vi "Lift Safety.vi"(11 "Operation States":T2) -> (3 "Operation States Out":T2)   [LabVIEW 2014]
uses:
  <vilib>/Rock Robotics/WPI/Solenoid/WPI_SolenoidValue.ctl
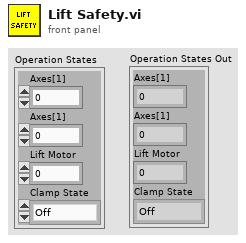
[diagram p1: front panel]
types:
  T1 = typedef "WPI_SolenoidValue.ctl" = enum16{"Off", "On", "Forward", "Reverse"}
  T2 = cluster{"Axes[1]":dbl, "Axes[1]":dbl, "Lift Motor":dbl, "Clamp State":T1}
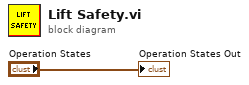
[diagram p0: block diagram]
diagram:
  "Operation States Out" <- "Operation States"
